vi "bats.parser.runHostToFpgaTests.vi"() -> (3 "All Passed?":bool)   [LabVIEW 2022 SP3]
panel:
  out "Results":cluster{"Test Name":string, "Passed?":bool}[](array[cluster])
  out "# of Passed Tests":i32
  out "Seconds":u32
  out "Minutes":u32
  out "# of Test Results":i32
  out "Get All Control\nValues Variant":T1(array[cluster])
  out "error out":errorcluster
  in  "error in":errorcluster
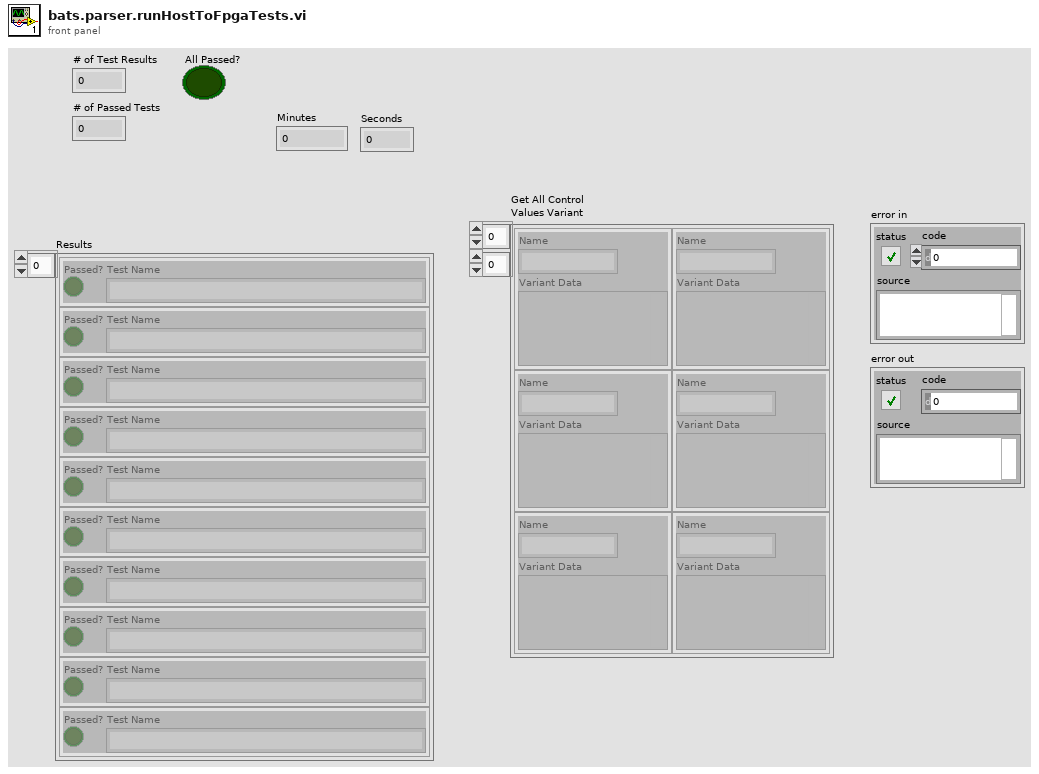
[diagram p1: front panel]
types:
  T1 = cluster{"Name":string, "Variant Data":variant}[][]
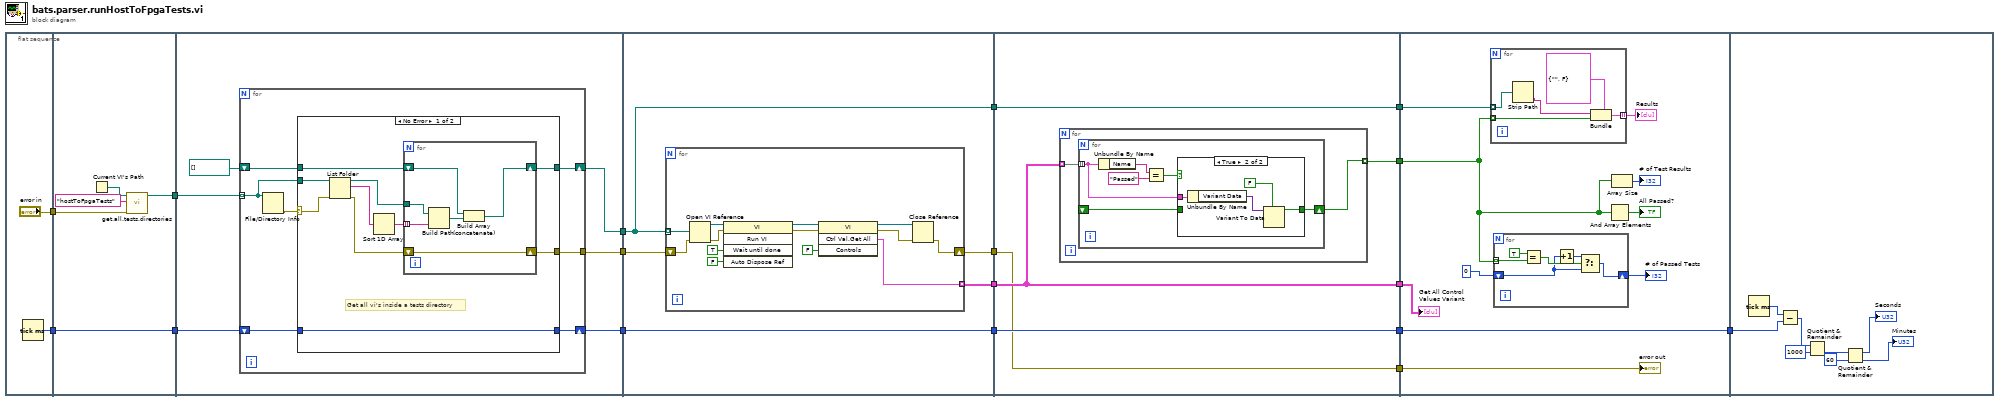
[diagram p0: block diagram]
diagram:
  n1 = flat-sequence {
    tunnel: [w19] -> w16
    tunnel: ["error in"] -> w9
    tunnel: [w24] -> w17
    tunnel: w16 -> [w24]
    tunnel: w9 -> [w21]
    tunnel: [w22] -> w8
    tunnel: w17 -> [w28]
    tunnel: [w30] -> w7
    tunnel: [w29] -> w3
    tunnel: w8 -> [w27]
    tunnel: [w25] -> w1
    tunnel: w7 -> [w58]
    tunnel: [w59] -> w6
    tunnel: [w60] -> w5
    tunnel: [w57] -> w4
    tunnel: w3 -> [w61]
    tunnel: [w61] -> w2
    tunnel: w1 -> [w57]
    tunnel: w6 -> [w75]
    tunnel: w5 -> [w76]
    tunnel: w4 -> [w79]
    tunnel: w2 -> [w78]
    tunnel: [w79] -> w15
    tunnel: [w78] -> w14
    tunnel: [w77] -> w13
    tunnel: [w76] -> w12
    tunnel: [w75] -> w11
    tunnel: w15 -> [w100]
    tunnel: w14 -> [w102]
    tunnel: w13 -> [w96]
    tunnel: w12 -> [w101]
    tunnel: w11 -> [w97]
    tunnel: [w102] -> w10
    tunnel: w10 -> [w120]
    frame #0 {
      n2 = Tick Count (ms)() -> (millisecond timer value=w19:u32)
    }
    frame #1 {
      n3 = Current VI's Path() -> (path=w23:path)
      n4 = call "get.all.tests.directories.vi"("error in"=w21, "filter"="hostToFpgaTests", "Path.in"=w23) -> ("Test Directories"=w22:path[])  [unwired: 7 in, 1 out]
    }
    frame #2 {
      n5 = for {
        tunnel: [w37] -> w30
        shift-right: [w36] -> w29
        shift-left: w28 -> [w35]
        tunnel: w27 -> [w33] mode=indexing
        shift-right: [w31] -> w25
        shift-left: path[] [] -> [w32]
        n6 = File/Directory Info(path=w33) -> (error out=w34:errorcluster)  [unwired: 1 in, 6 out]
        n7 = case shown="No Error" w34 {
          selector: w34 -> [w46 w56]
          tunnel: w33 -> [w47 _]
          tunnel: [w43 w56] -> w37
          tunnel: w35 -> [w42 w55]
          tunnel: [w42 w55] -> w36
          tunnel: [w39 w54] -> w31
          tunnel: w32 -> [w38 w54]
          frame No Error {
            # "Get all vi's inside a tests directory"
            n8 = List Folder(path=w47, error in=w46) -> (path out=w45:path, filenames=w41:string[], error out=w44:errorcluster)  [unwired: 2 in, 1 out]
            n9 = Sort 1D Array(array=w41) -> (sorted array=w40:string[])
            n10 = for {
              tunnel: w45 -> [w53]
              shift-right: [w48] -> w43
              shift-left: w44 -> [w48]
              tunnel: w40 -> [w52] mode=indexing
              shift-right: [w50] -> w39
              shift-left: w38 -> [w49]
              n11 = Build Path(base path=w53, name or relative path=w52) -> (appended path=w51:path)
              n12 = Build Array (concatenate)(w49, w51) -> (w50:path[])
            }
          }
          frame Error {
          }
        }
      }
    }
    frame #3 {
      n13 = for {
        tunnel: [w65] -> w60 mode=indexing
        tunnel: w57 -> [w64] mode=indexing
        shift-right: [w63] -> w59
        shift-left: w58 -> [w62]
        n14 = Open VI Reference(vi path=w64, error in (no error)=w62) -> (vi reference=w74:refnum<vi>, error out=w73:errorcluster)  [unwired: 4 in]
        n15 = invoke class="VI" method="Run VI"(reference=w74, error in=w73, "Wait until done"=TRUE ("Wait Until Done"), "Auto Dispose Ref"=FALSE ("Auto Dispose Reference")) -> (reference out=w72:refnum<vi>, error out=w67:errorcluster)  [unwired: 1 in, 3 out]
        n16 = invoke class="VI" method="Ctrl Val.Get All"(reference=w72, error in=w67, "Controls"=FALSE) -> (reference out=w68:refnum<vi>, error out=w66:errorcluster, "Get All Control Values Variant"=w65:cluster{"Name":string, "Variant Data":variant}[])  [unwired: 1 in, 1 out]
        n17 = Close Reference(reference=w68, error in (no error)=w66) -> (error out=w63:errorcluster)
      }
    }
    frame #4 {
      n18 = for {
        tunnel: w76 -> [w81] mode=indexing
        tunnel: [w80] -> w77 mode=indexing
        n19 = for {
          tunnel: w81 -> [w84] mode=indexing
          shift-right: [w83] -> w80
          shift-left: _ -> [w82]
          n20 = Unbundle By Name(w84) -> ("Name"=w87:string)
          n21 = Equal?(x=w87, y="Passed") -> (x = y?=w85:bool)
          n22 = case shown="True" w85 {
            tunnel: w84 -> [_ w92]
            tunnel: [w88 w89] -> w83
            tunnel: w82 -> [w88 _]
            frame False {
            }
            frame True {
              n23 = Unbundle By Name(w92) -> ("Variant Data"=w91:variant)
              n24 = Variant To Data(type=FALSE, Variant=w91) -> (data=w89:bool)  [unwired: 1 in, 1 out]
            }
          }
        }
      }
    }
    frame #5 {
      n25 = for {
        tunnel: w100 -> [w110] mode=indexing
        tunnel: w96 -> [w113] mode=indexing
        tunnel: [w112] -> w93 mode=indexing
        n26 = Strip Path(path=w110) -> (name=w109:string)  [unwired: 1 out]
        n27 = Bundle(cluster=cluster{"Test Name":string, "Passed?":bool} {"Test Name"="", "Passed?"=FALSE}, "Test Name"=w109, "Passed?"=w113) -> (w112:cluster{"Test Name":string, "Passed?":bool})
      }
      "Results" <- w93
      n28 = for {
        tunnel: w96 -> [w108] mode=indexing
        shift-right: [w105] -> w94
        shift-left: 0 -> [w104]
        n29 = Equal?(x=TRUE, y=w108) -> (x = y?=w106:bool)
        n30 = Increment(x=w104) -> (x+1=w103:i32)
        n31 = Select(t=w103, s=w106, f=w104) -> (s? t:f=w105:i32)
      }
      "# of Passed Tests" <- w94
      n32 = And Array Elements(Boolean array=w96) -> (logical AND=→"All Passed?":bool)
      n33 = Array Size(array=w96) -> (size(s)=→"# of Test Results":i32)
      "Get All Control\nValues Variant" <- w101
      "error out" <- w97
    }
    frame #6 {
      n34 = Tick Count (ms)() -> (millisecond timer value=w121:u32)
      n35 = Subtract(x=w121, y=w120) -> (x-y=w119:u32)
      n36 = Quotient & Remainder(x=w119, y=u32 1000) -> (floor(x/y)=w117:u32)  [unwired: 1 out]
      n37 = Quotient & Remainder(x=w117, y=u32 60) -> (x-y*floor(x/y)=→"Seconds":u32, floor(x/y)=→"Minutes":u32)
    }
  }
